vi "Write Orientation.vi"(8 "error in (no error)":errorcluster, 10 "Orientation":dbl[](array[numeric]), 11 "GoToSkill in":refnum<class "GoToSkill.lvclass">) -> (0 "error out":errorcluster, 3 "GoToSkill out":refnum<class "GoToSkill.lvclass">)   [LabVIEW 2022 SP3, in "GoToSkill.lvclass"]
uses:
  GoToSkill.lvclass
  GoToSkill.lvclass/GoToSkill.ctl
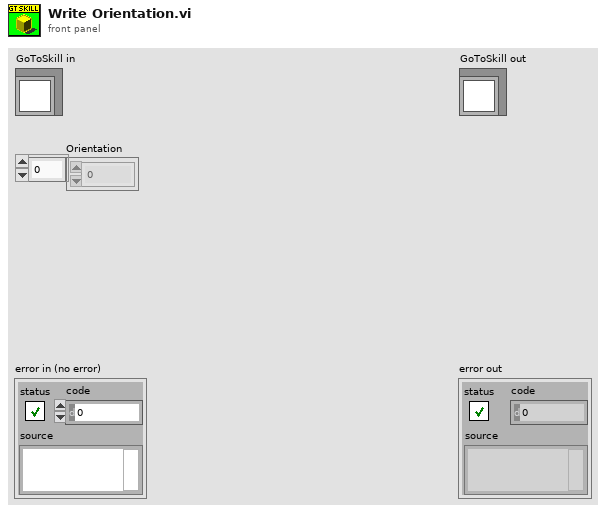
[diagram p1: front panel]
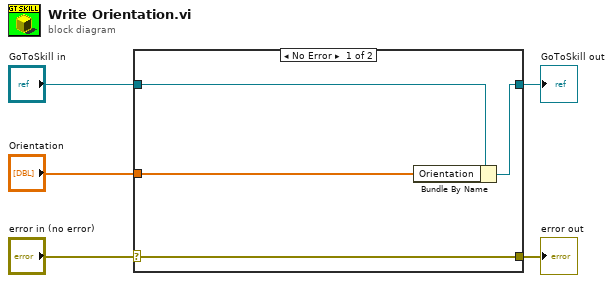
[diagram p0: block diagram]
diagram:
  n1 = case shown="No Error" "error in (no error)" {
    selector: "error in (no error)" -> [w9 w10]
    tunnel: [w9 w10] -> w4
    tunnel: [w7 w11] -> w2
    tunnel: "GoToSkill in" -> [w8 w11]
    tunnel: "Orientation" -> [w6 _]
    frame No Error {
      n2 = Bundle By Name(cluster=w8, "Orientation"=w6) -> (w7:refnum<class "GoToSkill.lvclass">)
    }
    frame Error {
    }
  }
  "error out" <- w4
  "GoToSkill out" <- w2
